vi "CT UDP.vi"() -> ()   [LabVIEW 2010]
panel:
  in  "Text":string
  out "Sensores":string
  out "A 2":bool
  out "B 2":bool
  in  "stop 2":bool
  in  "B":bool
  in  "A":bool
  in  "stop":bool
  # "Envio UDP"
  # "Recepcion UDP"
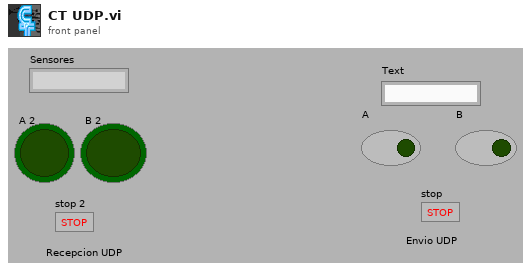
[diagram p1: front panel]
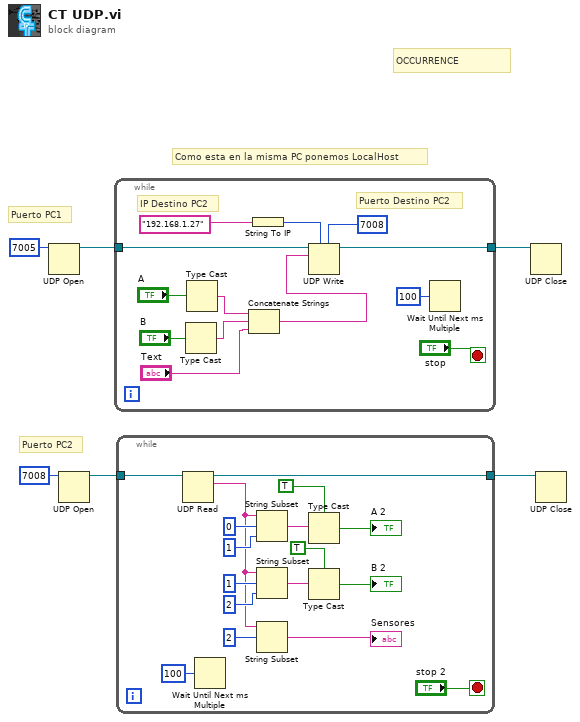
[diagram p0: block diagram]
diagram:
  # "Puerto PC2"
  # "Como esta en la misma PC ponemos LocalHost"
  # "Puerto PC1"
  # "OCCURRENCE"
  n1 = UDP Open(11:u16 7005 ("port")) -> (port=w6:refnum<k16>)  [unwired: 4 in, 2 out]
  n2 = UDP Open(11:u16 7008 ("port")) -> (port=w3:refnum<k16>)  [unwired: 4 in, 2 out]
  n3 = while {
    tunnel: w6 -> [w19]
    tunnel: [w18] -> w5
    stop <- "stop" stop-if-true
    # "IP Destino PC2"
    # "Puerto Destino PC2"
    n4 = Type Cast(x="B") -> (*(type *) &x=w11:string)  [unwired: 1 in]
    n5 = Type Cast(x="A") -> (*(type *) &x=w12:string)  [unwired: 1 in]
    n6 = Concatenate Strings "Concatenate Strings"(w12, w11, "Text") -> (w10:string)
    n7 = String To IP(1:"192.168.1.27" ("name")) -> (0:w15:u32)
    n8 = UDP Write(address=w15, port or service name=u16 7008, connection ID=w19, data in=w10) -> (3:w18:refnum<k16>)  [unwired: 2 in, 1 out]
    n9 = Wait Until Next ms Multiple(millisecond multiple=u32 100) -> ()  [unwired: 1 out]
  }
  n10 = while {
    tunnel: w3 -> [w36]
    tunnel: [w35] -> w2
    stop <- "stop 2" stop-if-true
    n11 = UDP Read(connection ID=w36) -> (data out=w22:string, 3:w35:refnum<k16>)  [unwired: 3 in, 3 out]
    n12 = Wait Until Next ms Multiple(millisecond multiple=u32 100) -> ()  [unwired: 1 out]
    n13 = String Subset(string=w22, offset (0)=0, length (rest)=1 ("offset (0)")) -> (substring=w30:string)
    n14 = String Subset(string=w22, offset (0)=1, length (rest)=2 ("offset (0)")) -> (substring=w29:string)
    n15 = String Subset(string=w22, offset (0)=2) -> (substring=→"Sensores":string)  [unwired: 1 in]
    n16 = Type Cast(type=TRUE, x=w30) -> (*(type *) &x=→"A 2":bool)
    n17 = Type Cast(type=TRUE, x=w29) -> (*(type *) &x=→"B 2":bool)
  }
  n18 = UDP Close(connection ID=w5) -> ()  [unwired: 1 in, 2 out]
  n19 = UDP Close(connection ID=w2) -> ()  [unwired: 1 in, 2 out]
